vi "Maths.vi"(6 "Curseur tracé":i32, 8 "Indice curseur 2":i32, 9 "Indice curseur 1":i32, 10 "Graphe":T1(graph)) -> (2 "Calculs maths":dbl[](array[numeric]))   [LabVIEW 2013]
uses:
  <vilib>/Analysis/8numeric.llb/1D Numeric Integration.vi
  <vilib>/Analysis/NI_AALBase.lvlib
  <vilib>/Analysis/NI_AALPro.lvlib
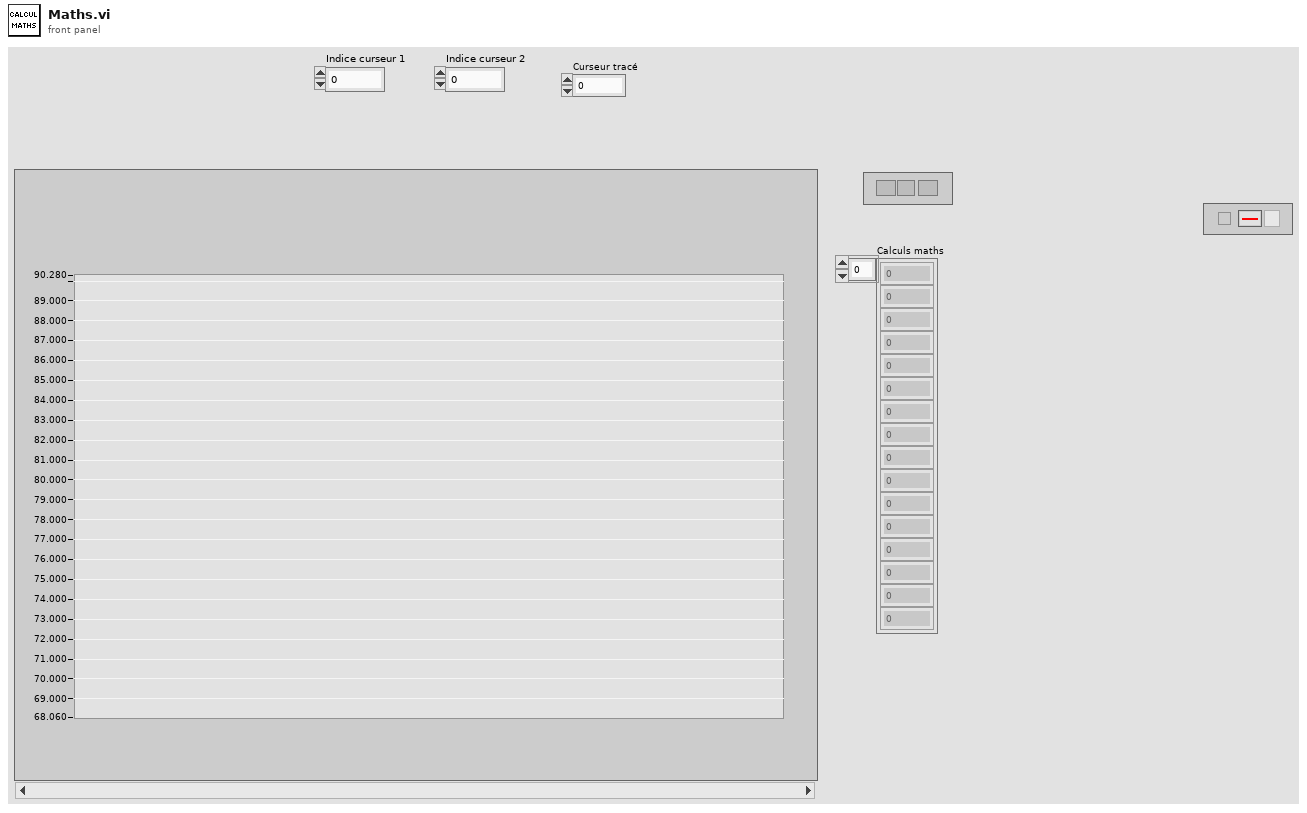
[diagram p1: front panel]
types:
  T1 = cluster{"Horodatage":timestamp[], "Donnees":dbl[]}[]
  T2 = cluster{"Horodatage":timestamp[], "Donnees":dbl[]}
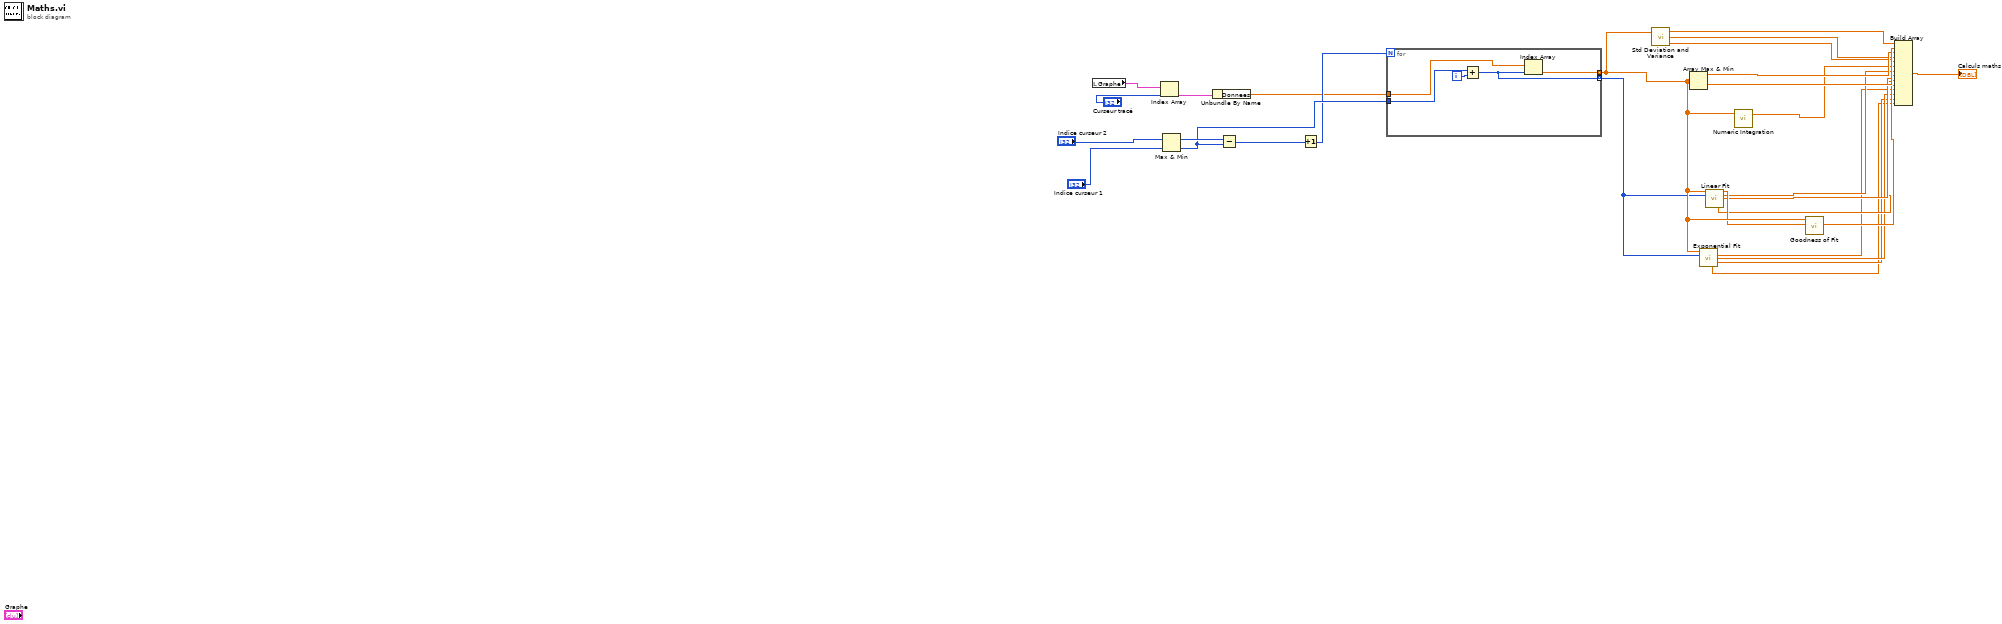
[diagram p0: block diagram]
diagram:
  n1 = local read "Graphe"() -> (w24:T1)
  n2 = Index Array(array=w24, index="Curseur tracé") -> (element=w23:T2)
  n3 = Max & Min(x="Indice curseur 2", y="Indice curseur 1") -> (max(x,y)=w28:i32, min(x,y)=w27:i32)
  n4 = Unbundle By Name(w23) -> ("Donnees"=w21:dbl[])
  n5 = Subtract(x=w28, y=w27) -> (x-y=w26:i32)
  n6 = Increment(x=w26) -> (x+1=w25:i32)
  n7 = for {
    N: w25 -> [_]
    tunnel: w27 -> [w33]
    tunnel: w21 -> [w31]
    tunnel: [w30] -> w18 mode=indexing
    tunnel: [w29] -> w16 mode=indexing
    i -> [w32]
    n8 = Add(x=w33, y=w32) -> (x+y=w29:i32)
    n9 = Index Array(array=w31, index=w29) -> (element=w30:dbl)
  }
  n10 = call <vilib>:"Std Deviation and Variance.vi"("X"=w18) -> ("mean"=w15:dbl, "standard deviation"=w12:dbl, "variance"=w11:dbl)  [unwired: 1 in]
  n11 = Array Max & Min(array=w18) -> (max value=w13:dbl, min value=w14:dbl)  [unwired: 2 out]
  n12 = call <vilib>:"Exponential Fit.vi"("Y"=w18, "X"=w16) -> ("amplitude"=w5:dbl, "damping"=w4:dbl, "offset"=w3:dbl, "residue"=w2:dbl)  [unwired: 8 in, 2 out]
  n13 = call <vilib>:"Linear Fit.vi"("Y"=w18, "X"=w16) -> ("Best Linear Fit"=w17:dbl[], "slope"=w9:dbl, "intercept"=w8:dbl, "residue"=w7:dbl)  [unwired: 9 in, 1 out]
  n14 = call-poly <vilib>:"Numeric Integration.vi"("Input Array"=w18) -> ("result"=w10:dbl)  [unwired: 2 in, 1 out]
  n15 = call <vilib>:"Goodness of Fit.vi"("Best Fit"=w17, "Y"=w18) -> ("R-square"=w6:dbl)  [unwired: 6 in, 3 out]
  n16 = Build Array(w15, w14, w13, w12, w11, w10, w9, w8, w7, w6, w5, w4, w3, w2) -> (→"Calculs maths":dbl[])
